vi "Has_Start_End.vi"(1 "Command":cluster{string, string[], dbl[], dbl}) -> (0 "Has Start and End":bool)   [LabVIEW 2011]
doc: "This VI examines a command and returns whether it has both \"Start\" and \"End\" variants."
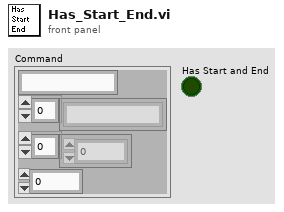
[diagram p1: front panel]
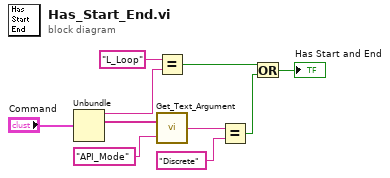
[diagram p0: block diagram]
diagram:
  n1 = Unbundle("Command") -> (w8:string, w3:string[])  [unwired: 2 out]
  n2 = Equal?(x="L_Loop", y=w8) -> (x = y?=w7:bool)
  n3 = call "Get_Text_Argument.vi"("Argument"="API_Mode", "Argument List"=w3) -> ("Text"=w2:string)
  n4 = Equal?(x=w2, y="Discrete") -> (x = y?=w6:bool)
  n5 = Or(x=w7, y=w6) -> (x .or. y?=→"Has Start and End":bool)
